vi "Example.vi"() -> ()   [LabVIEW 2015]
uses:
  Connect Channels (Single).vi
  Disconnect Channels (Single).vi
  SLSC Switch.lvclass
panel:
  in  "Topology":string
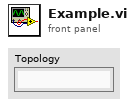
[diagram p1: front panel]
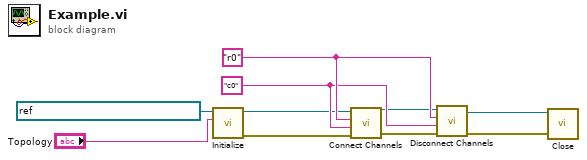
[diagram p0: block diagram]
diagram:
  w7 = "c0" ("channel 2")
  w8 = "r0" ("channel 1")
  n1 = call "Initialize.vi"("Topology"="Topology", "device"=refnum<k21> "SLSC-12001-030DA78A-Mod2") -> ("error out"=w5:errorcluster, "SLSC Switch out"=w6:refnum<class "SLSC Switch.lvclass">)  [unwired: 8 in]
  n2 = call-poly "Connect Channels.vi"("error in (no error)"=w5, "channel 2"=w7, "channel 1"=w8, "SLSC Switch in"=w6) -> ("error out"=w4:errorcluster, "SLSC Switch out"=w3:refnum<class "SLSC Switch.lvclass">)  [unwired: 6 in]
  n3 = call-poly "Disconnect Channels.vi"("error in (no error)"=w4, "channel 2"=w7, "channel 1"=w8, "SLSC Switch in"=w3) -> ("error out"=w1:errorcluster, "SLSC Switch out"=w2:refnum<class "SLSC Switch.lvclass">)  [unwired: 6 in]
  n4 = call "Close.vi"("error in (no error)"=w1, "SLSC Switch in"=w2) -> ()  [unwired: 9 in, 1 out]
